vi "GlobalBallHandling.vi"() -> ()   [LabVIEW 2023]
panel:
  out "OUT_Indexer_Beambreak":bool
  out "OUT_Shooter_Beambreak":bool
  out "OUT_ Intaking":bool
  out "OUT_Indexer_Shooter":dbl
  out "REF_Indexer_Shooter":string
  out "OUT_Indexer":dbl
  out "REF_Indexer":string
  out "REF_Rotator":string
  out "OUT_Rotator":dbl
  out "OUT_Intake":dbl
  out "REF_Intake":string
  # "DEVICE REFERENCE NAMES"
  # "Outputs"
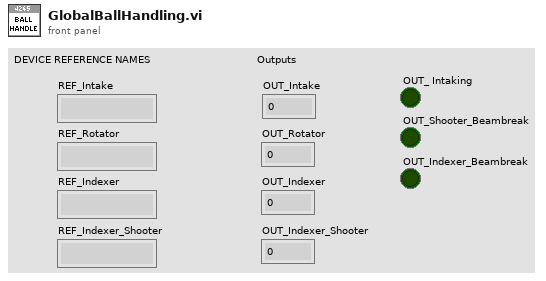
[diagram p1: front panel]
diagram:
